vi "thermo_format_units_all.vi"() -> (0 "all units":string[](array[string]), 1 "all tags":string[](array[string]), 2 "units":string[](array[string]), 3 "tags":string[](array[string]), 4 "count":i32)   [LabVIEW 2013]
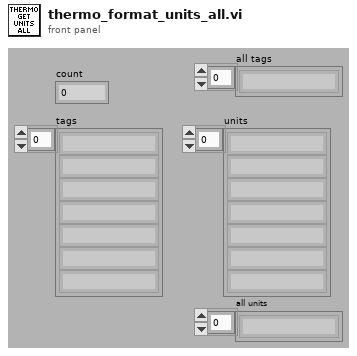
[diagram p1: front panel]
types:
  T1 = typedef "thermo.ctl" = cluster{"stat":enum16{"Disabled", "Enabled"}, "type":T2, "comment":string, "tag":string, "refresh":dbl, "IP":string, "port":u16, "VISA":refnum<visa-resource-name>, "last readout":timestamp, "TCP ref":refnum<k5>, "VISA sess":refnum<visa-resource-name>, "idn":string, "press":dbl, "RH":dbl, "temp":dbl, "pres cor":dbl[][], "RH cor":dbl[][], "temp cor":dbl[][], "try left":i32, "failed":bool, "RTD set":dbl[], "RTD inv":dbl[], "range":dbl, "net mode":enum16{"MODBUS", "HTTP"}}
  T2 = typedef "thermo_types.ctl" = enum16{"COMET Tx5xx (ethernet)", "Keithley 2002 (GPIB) + RTD", "Agilent 344xx (GPIB) + RTD"}
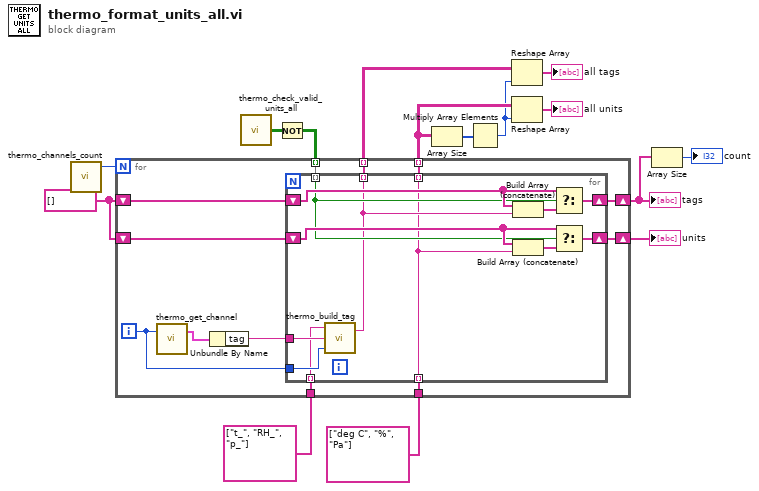
[diagram p0: block diagram]
diagram:
  w9 = string[] []
  n1 = call "thermo_channels_count.vi"() -> ("channels"=w15:i32)  [unwired: 2 in]
  n2 = call "thermo_check_valid_units_all.vi"() -> ("valids 2D"=w12:bool[][])  [unwired: 2 out]
  n3 = Not(x=w12) -> (.not. x?=w11:bool[][])
  n4 = for {
    N: w15 -> [_]
    shift-right: [w22] -> w8
    shift-left: w9 -> [w21]
    tunnel: w11 -> [w20] mode=indexing
    tunnel: string[] ["t_", "RH_", "p_"] -> [w24]
    tunnel: string[] ["deg C", "%", "Pa"] -> [w23]
    shift-right: [w18] -> w10
    shift-left: w9 -> [w19]
    tunnel: [w17] -> w6 mode=indexing
    tunnel: [w16] -> w5 mode=indexing
    i -> [w25]
    n5 = call "thermo_get_channel.vi"("index"=w25) -> ("channel"=w27:T1)  [unwired: 1 in, 1 out]
    n6 = Unbundle By Name(w27) -> ("tag"=w26:string)
    n7 = for {
      tunnel: w26 -> [w39]
      tunnel: w25 -> [w38]
      tunnel: w24 -> [w37] mode=indexing
      tunnel: w23 -> [w28] mode=indexing
      shift-right: [w36] -> w22
      shift-left: w21 -> [w34]
      tunnel: w20 -> [w30] mode=indexing
      shift-right: [w31] -> w18
      shift-left: w19 -> [w33]
      tunnel: [w29] -> w17 mode=indexing
      tunnel: [w28] -> w16 mode=indexing
      n8 = call "thermo_build_tag.vi"("index"=w38, "tag in"=w39, "tag prefix"=w37) -> ("merged tag out"=w29:string)  [unwired: 1 in, 1 out]
      n9 = Build Array (concatenate)(w34, w29) -> (w35:string[])
      n10 = Build Array (concatenate)(w33, w28) -> (w32:string[])
      n11 = Select(t=w34, s=w30, f=w35) -> (s? t:f=w36:string[])
      n12 = Select(t=w33, s=w30, f=w32) -> (s? t:f=w31:string[])
    }
  }
  "tags" <- w8
  "units" <- w10
  n13 = Array Size(array=w5) -> (size(s)=w4:i32[])
  n14 = Multiply Array Elements(1:w4) -> (0:w3:i32)
  n15 = Reshape Array(w6, w3) -> (→"all tags":string[])
  n16 = Reshape Array(w5, w3) -> (→"all units":string[])
  n17 = Array Size(array=w8) -> (size(s)=→"count":i32)
